vi "(SubVI) Five-Type Smooth Filters_YCC.vi"(3 "Filter type":T1(ring), 4 "Avg points":i32, 5 "Sampling rate (Hz)":dbl=20000.0, 6 "QPD data":dbl[](array[numeric])) -> (1 "Sampling rate after filtering (Hz)":dbl, 2 "Filtered QPD data":dbl[](array[numeric]))   [LabVIEW 2014]
uses:
  <vilib>/Analysis/3filter.llb/Savitzky-Golay Filter (DBL).vi
  <vilib>/Analysis/NI_AALBase.lvlib
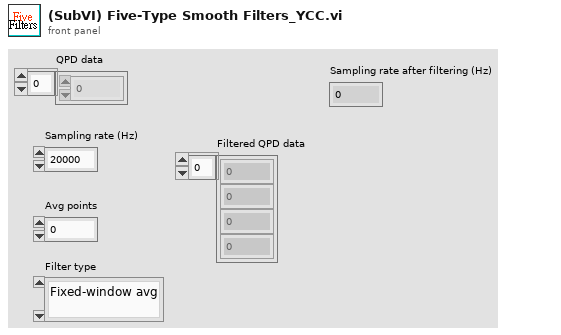
[diagram p1: front panel]
types:
  T1 = enum16{"Fixed-window avg", "Moving-window avg", "F+S-window avg", "S-G filter", "Fixed-window Median", "Moving-window Median "}
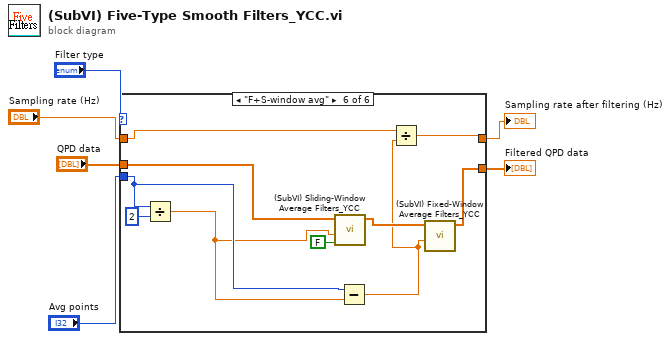
[diagram p0: block diagram]
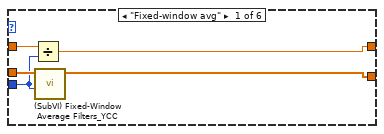
[diagram p2: hidden frame]
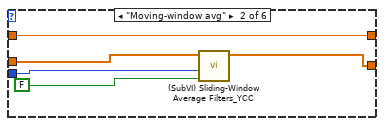
[diagram p3: hidden frame]
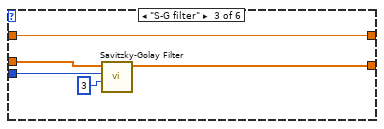
[diagram p4: hidden frame]
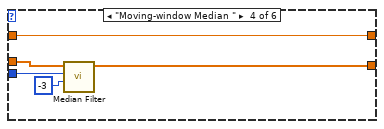
[diagram p5: hidden frame]
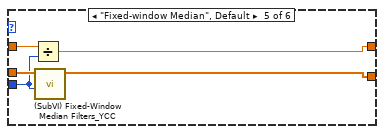
[diagram p6: hidden frame]
diagram:
  n1 = case shown="\"F+S-window avg\"" "Filter type" {
    tunnel: "Avg points" -> [w8 w15 w21 w26 w28 w38]
    tunnel: [w7 w14 w19 w24 w27 w35] -> w5
    tunnel: "QPD data" -> [w9 w13 w18 w23 w29 w39]
    tunnel: "Sampling rate (Hz)" -> [w11 w16 w17 w22 w31 w33]
    tunnel: [w10 w16 w17 w22 w30 w32] -> w3
    frame "Fixed-window avg" {
      n2 = Divide(x=w11, y=w8) -> (x/y=w10:dbl)
      n3 = call "(SubVI) Fixed-Window Average Filters_YCC.vi"("Avg points"=w8, "Signal"=w9) -> ("Filtered Signal"=w7:dbl[])  [unwired: 5 in]
    }
    frame "Moving-window avg" {
      n4 = call "(SubVI) Sliding-Window Average Filters_YCC.vi"("All add in the tail?"=FALSE, "Avg points"=w15, "Signal"=w13) -> ("Filtered Signal"=w14:dbl[])  [unwired: 4 in]
    }
    frame "S-G filter" {
      n5 = call-poly <vilib>:"Savitzky-Golay Filter.vi"("polynomial order"=3, "side points"=w21, "X"=w18) -> ("Filtered X"=w19:dbl[])  [unwired: 7 in, 1 out]
    }
    frame "Moving-window Median " {
      n6 = call <vilib>:"Median Filter.vi"("right rank"=-3, "left rank"=w26, "X"=w23) -> ("Filtered X"=w24:dbl[])  [unwired: 7 in, 1 out]
    }
    frame "Fixed-window Median", Default {
      n7 = Divide(x=w31, y=w28) -> (x/y=w30:dbl)
      n8 = call "(SubVI) Fixed-Window Median Filters_YCC.vi"("Avg points"=w28, "Signal"=w29) -> ("Filtered Signal"=w27:dbl[])  [unwired: 5 in]
    }
    frame "F+S-window avg" {
      n9 = Divide(x=w38, y=2) -> (x/y=w37:dbl)
      n10 = call "(SubVI) Sliding-Window Average Filters_YCC.vi"("All add in the tail?"=FALSE, "Avg points"=w37, "Signal"=w39) -> ("Filtered Signal"=w36:dbl[])  [unwired: 4 in]
      n11 = Subtract(x=w38, y=w37) -> (x-y=w34:dbl)
      n12 = Divide(x=w33, y=w34) -> (x/y=w32:dbl)
      n13 = call "(SubVI) Fixed-Window Average Filters_YCC.vi"("Avg points"=w34, "Signal"=w36) -> ("Filtered Signal"=w35:dbl[])  [unwired: 5 in]
    }
  }
  "Sampling rate after filtering (Hz)" <- w3
  "Filtered QPD data" <- w5
